vi "Shutdown.vi"(8 "error in (no error)":errorcluster, 10 "timeout_ms":i32=1000, 11 "Logger in":refnum<class "Logger.lvclass">) -> (0 "error out":errorcluster)   [LabVIEW 2026, in "Lumberjack.lvlib" / "Logger.lvclass"]
doc: "Stops the logging system and blocks until it is fully down. Sends the framework Stop to the LogManager, then waits on stoppedNotifier until the manager and all nested appenders have stopped (each having flushed and closed its sink). Runs its stop even if error in carries an error (SRS-LMBR-004). On a clean stop, merges the manager's exit error into error out; if the tree does not stop within timeout ms, returns error 5032. Releases both notifiers and clears the process-default logger before returning. Because it is synchronous, on return it is safe to reclaim application-owned resources such as relay queues. Control plane; not on the logging hot path."
uses:
  Logger.lvclass
  Logger.lvclass/Logger.ctl
  Lumberjack.lvlib
  Core/Messages/RequestShutdownMsg.lvclass/RequestShutdownMsg.lvclass
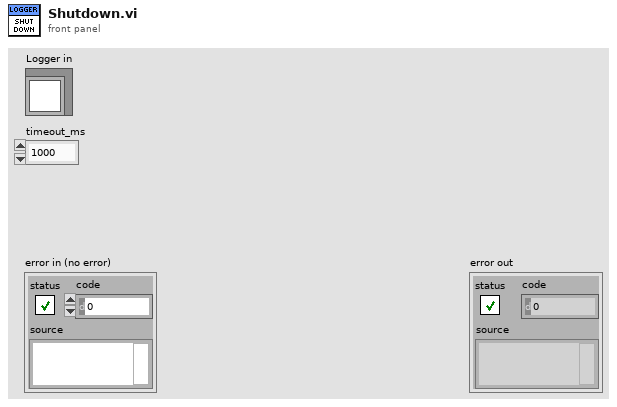
[diagram p1: front panel]
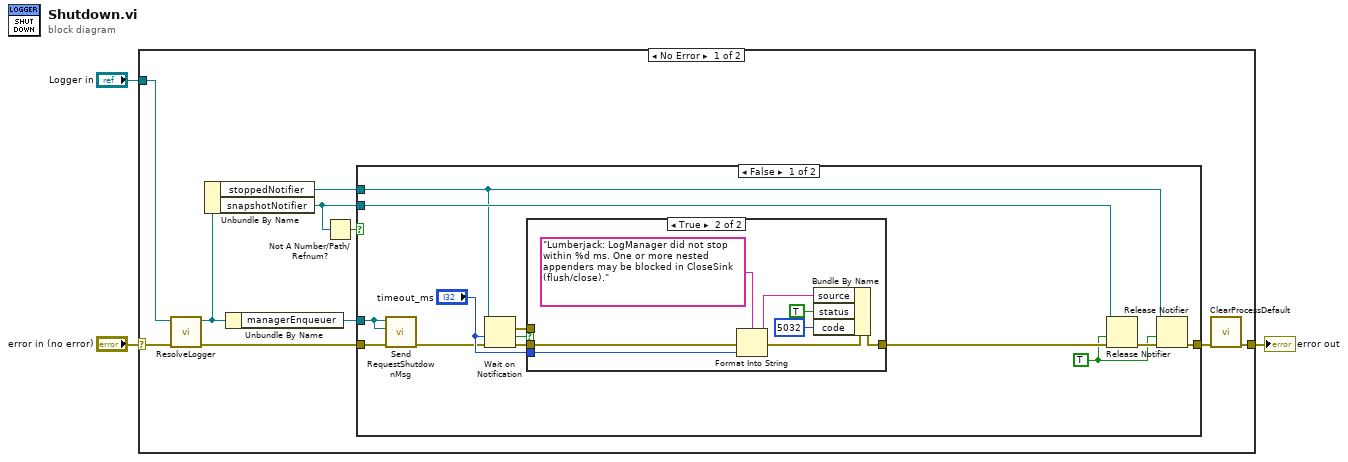
[diagram p0: block diagram]
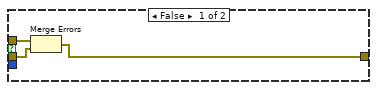
[diagram p2: hidden frame]
diagram:
  n1 = case shown="No Error" "error in (no error)" {
    selector: "error in (no error)" -> [w13 w39]
    tunnel: [w8 w39] -> w2
    tunnel: "Logger in" -> [w9 _]
    frame No Error {
      n2 = call "ResolveLogger.vi"("error in (no error)"=w13, "Logger in"=w9) -> ("error out"=w12:errorcluster, "Logger out"=w10:refnum<class "Logger.lvclass">)  [unwired: 8 in]
      n3 = Unbundle By Name(w10) -> ("stoppedNotifier"=w7:refnum<notifier>, "snapshotNotifier"=w5:refnum<notifier>)
      n4 = Unbundle By Name(w10) -> ("managerEnqueuer"=w4:refnum<class "Message Enqueuer.lvclass">)
      n5 = Not A Number/Path/Refnum?(number/path/refnum=w5) -> (NaN/Path/Refnum?=w11:bool)
      n6 = case shown="False" w11 {
        tunnel: w12 -> [w16 w38]
        tunnel: [w19 w38] -> w6
        tunnel: w7 -> [w18 _]
        tunnel: w5 -> [w22 _]
        tunnel: w4 -> [w15 _]
        frame False {
          w17 = TRUE ("force destroy? (F)")
          n7 = call "Send RequestShutdownMsg.vi"("error in (no error)"=w16, "enqueuer"=w15, "Enqueuer in"=w15) -> ("error out"=w14:errorcluster)  [unwired: 7 in, 1 out]
          n8 = Wait on Notification(notifier=w18, timeout in ms (-1)="timeout_ms", error in (no error)=w14) -> (notification=w23:errorcluster, timed out?=w24:bool, error out=w26:errorcluster)  [unwired: 1 in, 1 out]
          n9 = case shown="True" w24 {
            tunnel: w26 -> [w29 w34]
            tunnel: [w27 w31] -> w20
            tunnel: "timeout_ms" -> [_ w30]
            tunnel: w23 -> [w28 _]
            frame False {
              n10 = Merge Errors(w28, w29) -> (w27:errorcluster)
            }
            frame True {
              n11 = Format Into String(format string="Lumberjack: LogManager did not stop within %d ms. One or more nested appenders may be blocked in CloseSink (flush/close)." ("source"), error in=w34, w30) -> (resulting string=w37:string, error out=w36:errorcluster)  [unwired: 1 in]
              n12 = Bundle By Name(cluster=w36, "source"=w37, "status"=TRUE, "code"=5032) -> (w31:errorcluster)
            }
          }
          n13 = Release Notifier(notifier=w22, force destroy? (F)=w17, error in (no error)=w20) -> (error out=w21:errorcluster)  [unwired: 2 out]
          n14 = Release Notifier(notifier=w18, force destroy? (F)=w17, error in (no error)=w21) -> (error out=w19:errorcluster)  [unwired: 2 out]
        }
        frame True {
        }
      }
      n15 = call "ClearProcessDefault.vi"("error in (no error)"=w6) -> ("error out"=w8:errorcluster)  [unwired: 10 in]
    }
    frame Error {
    }
  }
  "error out" <- w2
